vi "Pre Launch Init.vi"(11 "Task in":refnum<class "Task.lvclass">) -> (0 "error out":errorcluster, 3 "Task out":refnum<class "Task.lvclass">)   [LabVIEW 2020, in "Volatus.lvlib" / "Task.lvclass"]
doc: "(<B>Filename</B>: Actor Framework.lvlib:Actor.lvclass:Pre Launch Init.vi)\n\nDefines behavior that occurs after the Launch Nested Actor method is invoked but before the actor's Actor Core method begins running.\n\nBy default, this method does nothing. A descendant class may override it to define behavior."
uses:
  Task.lvclass
  Task State.ctl
  Task.lvclass/Task.ctl
  Event API/EventAPI.lvclass/EventAPI.ctl
  EventHandler Messages/Handle Event Msg/Handle Event Msg.lvclass/Handle Event Msg.ctl
  <vilib>/ActorFramework/Message Enqueuer/Message Enqueuer.lvclass/Message Enqueuer.ctl
  Event API/Report Event.vi
  EventHandler Messages/Handle Event Msg/Send Handle Event.vi
  <vilib>/ActorFramework/Message Enqueuer/Enqueue.vi
  EventHandler Messages/Handle Event Msg/Handle Event Msg.lvclass
  C:/Program Files (x86)/National Instruments/LabVIEW 2020/vi.lib/ActorFramework/Message/Message.lvclass
  <vilib>/ActorFramework/Message Priority Queue/Priority Enqueue.vi
  Volatus.lvlib
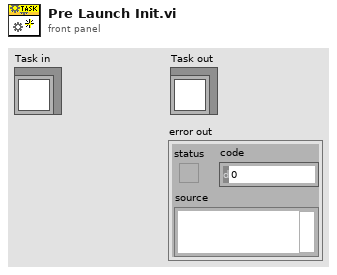
[diagram p1: front panel]
types:
  T1 = typedef "Volatus.lvlib/Task State.ctl" = enum16{"Unknown", "Idle", "Initializing", "Starting", "Running", "Stopping", "Stopped", "Error - Init", "Error - Start", "Error - Run", "Error - Stop"}
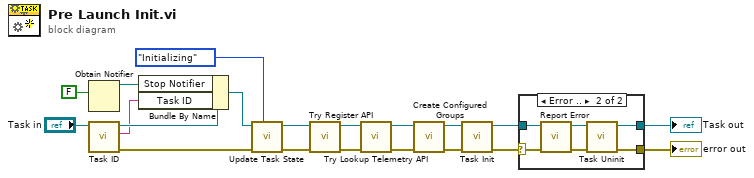
[diagram p0: block diagram]
diagram:
  n1 = Obtain Notifier(notification data type=FALSE) -> (notifier out=w6:refnum<notifier>)  [unwired: 3 in, 2 out]
  n2 = call-dynamic "Task ID.vi"("Task in"="Task in") -> ("error out"=w14:errorcluster, "Task ID"=w16:string, "Task out"=w17:refnum<class "Task.lvclass">)  [unwired: 8 in]
  n3 = Bundle By Name(cluster=w17, "Stop Notifier"=w6, "Task ID"=w16) -> (w15:refnum<class "Task.lvclass">)
  n4 = call "Update Task State.vi"("State"=Task_State."Initializing", "error in (no error)"=w14, "Task in"=w15) -> ("error out"=w13:errorcluster, "Task out"=w12:refnum<class "Task.lvclass">)  [unwired: 7 in]
  n5 = call "Try Register API.vi"("error in (no error)"=w13, "Task in"=w12) -> ("error out"=w11:errorcluster, "Task out"=w4:refnum<class "Task.lvclass">)  [unwired: 8 in]
  n6 = call "Try Lookup Telemetry API.vi"("error in (no error)"=w11, "Task in"=w4) -> ("error out"=w5:errorcluster, "Task out"=w2:refnum<class "Task.lvclass">)  [unwired: 8 in]
  n7 = call "Create Configured Groups.vi"("error in (no error)"=w5, "Task in"=w2) -> ("error out"=w3:errorcluster, "Task out"=w1:refnum<class "Task.lvclass">)  [unwired: 8 in]
  n8 = call-dynamic "Task Init.vi"("error in (no error)"=w3, "Task in"=w1) -> ("error out"=w20:errorcluster, "Task out"=w9:refnum<class "Task.lvclass">)  [unwired: 8 in]
  n9 = case shown="Error .." w20 {
    selector: w20 -> [w21 w28]
    tunnel: [w21 w27] -> w10
    tunnel: w9 -> [w22 w24]
    tunnel: [w22 w26] -> w8
    frame No Error {
    }
    frame Error {
      n10 = call "Report Error.vi"("error in (no error)"=w28, "Task in"=w24) -> ("error out"=w25:errorcluster, "Task out"=w23:refnum<class "Task.lvclass">)  [unwired: 8 in]
      n11 = call-dynamic "Task Uninit.vi"("error in (no error)"=w25, "Task in"=w23) -> ("error out"=w27:errorcluster, "Task out"=w26:refnum<class "Task.lvclass">)  [unwired: 8 in]
    }
  }
  "error out" <- w10
  "Task out" <- w8
